vi "Identify.vi"(8 "error in (no error)":errorcluster, 11 "QPA TCF Parser in":refnum<class "QPA TCF Parser.lvclass">) -> (0 "error out":errorcluster, 2 "Plugin is Valid":bool, 3 "QPA TCF Parser out":refnum<class "QPA TCF Parser.lvclass">)   [LabVIEW 2016, in "QPA TCF Parser.lvlib" / "QPA TCF Parser.lvclass"]
uses:
  QPA TCF Parser.lvclass
  C:/Projects/STS/Common/Sequence Automation/Plugins/File Parsing Interface.lvlibp/File Parsing Interface.lvclass
  Plugins/File Parsing Interface.lvlibp/Accessors/File to Parse/Read File to Parse.vi
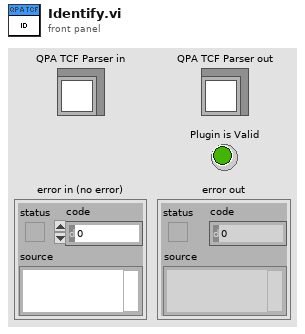
[diagram p1: front panel]
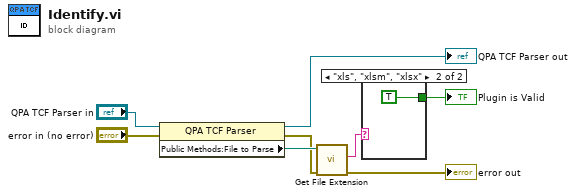
[diagram p0: block diagram]
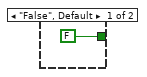
[diagram p2: hidden frame]
diagram:
  n1 = property class="QPA TCF Parser"(reference="QPA TCF Parser in", error in="error in (no error)") -> (reference out=→"QPA TCF Parser out":refnum<class "QPA TCF Parser.lvclass">, error out=w4:errorcluster, "Public Methods:File to Parse"=w5:path)
  n2 = call <vilib>:"Get File Extension.vi"("error in (no error)"=w4, "file"=w5) -> ("error out"=→"error out":errorcluster, "lowercase file extension"=w2:string)  [unwired: 5 in, 3 out]
  n3 = case shown="\"xls\", \"xlsm\", \"xlsx\"" w2 {
    tunnel: [FALSE TRUE] -> w1
    frame "False", Default {
    }
    frame "xls", "xlsm", "xlsx" {
    }
  }
  "Plugin is Valid" <- w1
